vi "Dereference.vi"(7 "Type Specifier":refnum<class>, 8 "error in (no error)":errorcluster, 11 "InstrPtr":refnum<class "InstrPtr.lvclass">) -> (0 "error out":errorcluster, 2 "Instrument out":refnum<class>, 3 "InstrPtr out":refnum<class "InstrPtr.lvclass">)   [LabVIEW 2017, in "InstrPtr.lvclass"]
doc: "Dereference: this \"checks out\" the object, which you can then mutate with the standard accessor methods for the class. All other programs will wait (block) on this method until you check the object back in.\n\nThe Type Specifier input is discarded, but it is needed for type detection as an attempt to automatically downcast the retrieved object."
uses:
  InstrPtr.lvclass
  InstrPtr.lvclass/InstrPtr.ctl
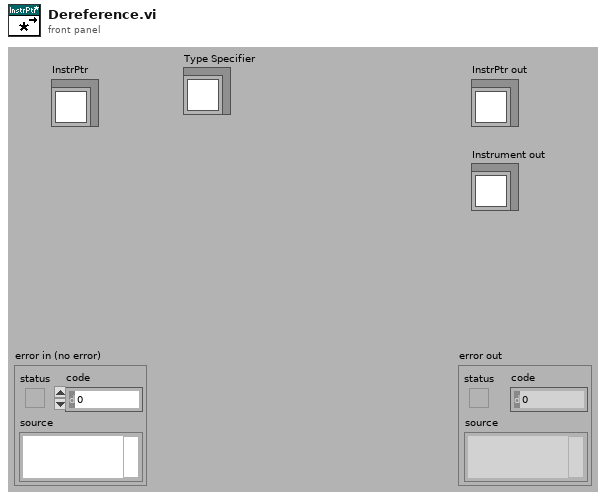
[diagram p1: front panel]
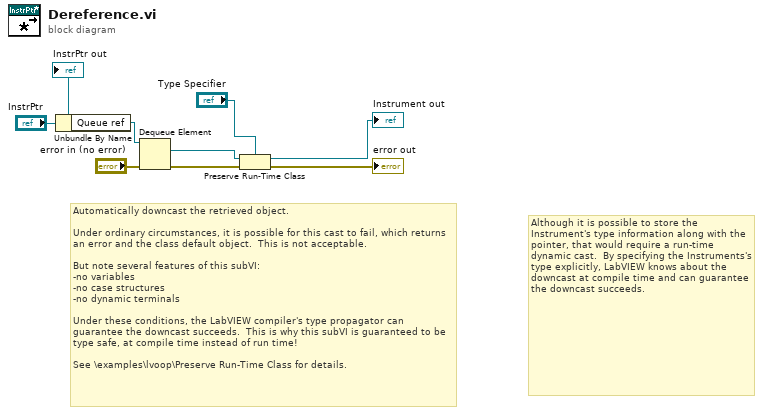
[diagram p0: block diagram]
diagram:
  # "Although it is possible to store the Instrument's type information along with the pointer, that would require a run-time dynamic cast.  By specifying the Instruments's type explicitly, LabVIEW knows about the downcast at compile time and can guarantee the downcast succeeds."
  # "Automatically downcast the retrieved object.\n\nUnder ordinary circumstances, it is possible for this cast to fail, which returns an error and the class default object.  This is not acceptable.\n\nBut note several features of this subVI:\n-no variables\n-no case structures\n-no dynamic terminals\n\nUnder these conditions, the LabVIEW compiler's type propagator can guarantee the downcast succeeds.  This is why this subVI is guaranteed to be type safe, at compile time instead of run time!\n\nSee \\examples\\lvoop\\Preserve Run-Time Class for details."
  n1 = Unbundle By Name("InstrPtr") -> ("Queue ref"=w5:refnum<queue>)
  n2 = Dequeue Element(queue=w5, error in (no error)="error in (no error)") -> (element=w4:refnum<class>, error out=w2:errorcluster)  [unwired: 3 out]
  n3 = Preserve Run-Time Class(object in=w4, error in=w2, 2:"Type Specifier") -> (object out=→"Instrument out":refnum<class>, error out=→"error out":errorcluster)
  "InstrPtr out" <- "InstrPtr"
